vi "MaquinaEstados.vi"() -> ()   [LabVIEW 2018]
uses:
  CaseEnum.ctl
panel:
  out "Ventilador Derecho":dbl(knob) scale=0.0..10.0
  out "Ventilador Izquierdo":dbl(knob) scale=0.0..10.0
  out "Estado Actual":T1
  in  "Termometro":dbl(slide) scale=0.0..200.0
  in  "stop":bool
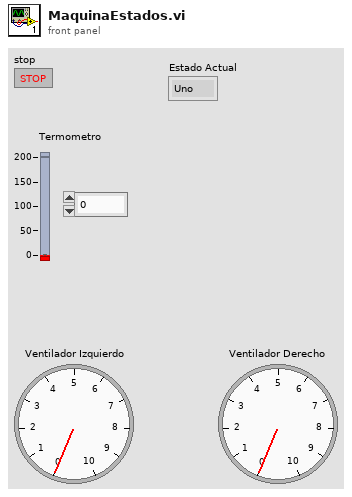
[diagram p1: front panel]
types:
  T1 = typedef "CaseEnum.ctl" = enum16{"Uno", "Dos", "Tres", "Cuatro", "Cinco", "Seis"}
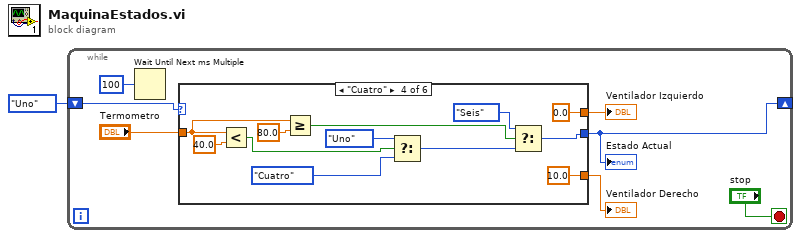
[diagram p0: block diagram]
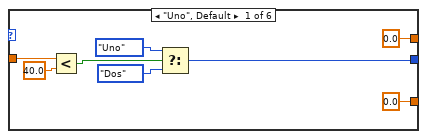
[diagram p2: hidden frame]
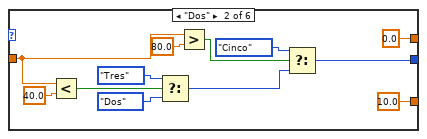
[diagram p3: hidden frame]
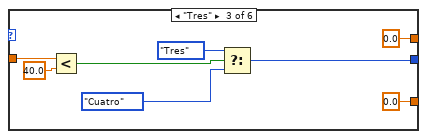
[diagram p4: hidden frame]
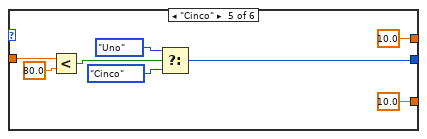
[diagram p5: hidden frame]
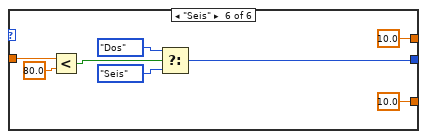
[diagram p6: hidden frame]
diagram:
  n1 = while {
    shift-right: [w4] -> _
    shift-left: CaseEnum."Uno" -> [w6]
    stop <- "stop" stop-if-true
    n2 = Wait Until Next ms Multiple(millisecond multiple=u32 100) -> ()  [unwired: 1 out]
    n3 = case shown="\"Cuatro\"" w6 {
      tunnel: "Termometro" -> [w16 w21 w34 w43 w56 w64]
      tunnel: [w11 w17 w31 w40 w51 w59] -> w4
      tunnel: [0.0 0.0 0.0 0.0 10.0 10.0] -> w3
      tunnel: [0.0 10.0 0.0 10.0 10.0 10.0] -> w2
      frame "Uno", Default {
        n4 = Less?(x=w16, y=40.0) -> (x < y?=w14:bool)
        n5 = Select(t=CaseEnum."Uno", s=w14, f=CaseEnum."Dos") -> (s? t:f=w11:T1)
      }
      frame "Dos" {
        n6 = Less?(x=w21, y=40.0) -> (x < y?=w18:bool)
        n7 = Select(t=CaseEnum."Tres", s=w18, f=CaseEnum."Dos") -> (s? t:f=w26:T1)
        n8 = Greater?(x=w21, y=80.0) -> (0:w24:bool)
        n9 = Select(t=CaseEnum."Cinco", s=w24, f=w26) -> (s? t:f=w17:T1)
      }
      frame "Tres" {
        n10 = Less?(x=w34, y=40.0) -> (x < y?=w35:bool)
        n11 = Select(t=CaseEnum."Tres", s=w35, f=CaseEnum."Cuatro") -> (s? t:f=w31:T1)
      }
      frame "Cuatro" {
        n12 = Less?(x=w43, y=40.0) -> (x < y?=w38:bool)
        n13 = Greater Or Equal?(x=w43, y=80.0) -> (x >= y?=w46:bool)
        n14 = Select(t=CaseEnum."Uno", s=w38, f=CaseEnum."Cuatro") -> (s? t:f=w48:T1)
        n15 = Select(t=CaseEnum."Seis", s=w46, f=w48) -> (s? t:f=w40:T1)
      }
      frame "Cinco" {
        n16 = Less?(x=w56, y=80.0) -> (x < y?=w54:bool)
        n17 = Select(t=CaseEnum."Uno", s=w54, f=CaseEnum."Cinco") -> (s? t:f=w51:T1)
      }
      frame "Seis" {
        n18 = Less?(x=w64, y=80.0) -> (x < y?=w62:bool)
        n19 = Select(t=CaseEnum."Dos", s=w62, f=CaseEnum."Seis") -> (s? t:f=w59:T1)
      }
    }
    "Estado Actual" <- w4
    "Ventilador Derecho" <- w2
    "Ventilador Izquierdo" <- w3
  }
